vi "Launch WaitAny helper.vi"(9 "Timeout":i32, 10 "Forwarded Event":refnum<user-event>, 11 "Event Reg":refnum<event-registration>) -> (0 "error out":errorcluster)   [LabVIEW 2020, in "Promises.lvlib" / "Future.lvclass"]
uses:
  Future.lvclass
  Result.ctl
  Result State.ctl
  WaitAny Helper Async.vi
  Promises.lvlib
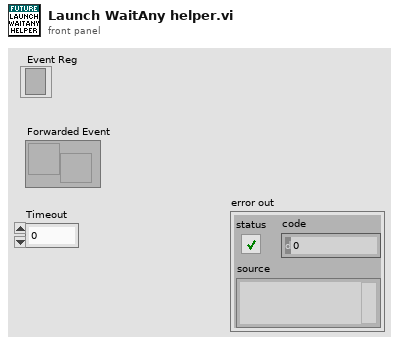
[diagram p1: front panel]
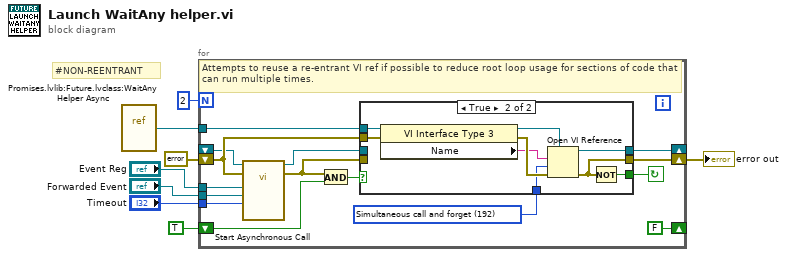
[diagram p0: block diagram]
diagram:
  # "#NON-REENTRANT"
  n1 = vi-ref "Promises.lvlib:Future.lvclass:WaitAny Helper Async.vi"() -> (w6:refnum<vi>)
  n2 = for {
    N: 2 -> [_]
    tunnel: w6 -> [w22]
    shift-right: [w21] -> _
    shift-left: _ -> [w20]
    shift-right: [w18] -> w2
    shift-left: errorcluster {"status"=FALSE, "code"=0, "source"=""} ("error constant") -> [w23]
    shift-right: [FALSE] -> _
    shift-left: TRUE -> [w15]
    tunnel: "Timeout" -> [w12]
    tunnel: "Forwarded Event" -> [w11]
    tunnel: "Event Reg" -> [w10]
    stop <- w14 continue-if-true
    w9 = 192 items=["Record modifications"=1, "Open templates for editing"=2, "Prompt user to save"=4, "Prepare for reentrant run"=8, "Prompt to find missing subVIs"=16, "Hide loading dialog box"=32, "Enable simultaneous calls"=64, "Prepare to call and forget"=128, "Simultaneous call and forget"=192, "Prepare to call and collect"=256, "Simultaneous call and collect"=320]
    # "Attempts to reuse a re-entrant VI ref if possible to reduce root loop usage for sections of code that can run multiple times."
    n3 = call-by-ref "Start Asynchronous Call"(reference=w20, error in=w23, "Timeout"=w12, "Forwarded Event"=w11, "Event Reg"=w10) -> (reference out=w19:refnum<vi>, error out=w17:errorcluster)  [unwired: 9 in]
    n4 = And(x=w17, y=w15) -> (x .and. y?=w16:bool)
    n5 = case shown="True" w16 {
      tunnel: w22 -> [_ w33]
      tunnel: w9 -> [_ w31]
      tunnel: [w25 w29] -> w21
      tunnel: w19 -> [w25 _]
      tunnel: [w24 w27] -> w18
      tunnel: w17 -> [w24 _]
      tunnel: w23 -> [_ w28]
      tunnel: [_ w26] -> w14
      frame False {
      }
      frame True {
        n6 = property class="VI Interface Type 3"(reference=w33, error in=w28) -> (reference out=w30:refnum<vi>, error out=w34:errorcluster, "Name"=w32:string)
        n7 = Open VI Reference(type specifier VI Refnum (for type only)=w30, vi path=w32, options=w31, error in (no error)=w34) -> (vi reference=w29:refnum<vi>, error out=w27:errorcluster)  [unwired: 2 in]
        n8 = Not(x=w27) -> (.not. x?=w26:bool)
      }
    }
  }
  "error out" <- w2
